vi "Robot Movement Command Interpreter-poly.vi"   [LabVIEW 2019]
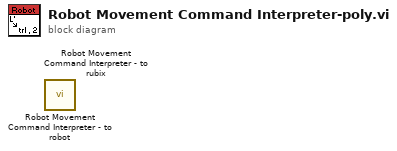
[diagram p0: block diagram]
diagram:
  n1 = call "Robot Movement Command Interpreter - to robot.vi"() -> ()  [unwired: 11 in, 1 out]
  n2 = call "Robot Movement Command Interpreter - to rubix.vi"() -> ()  [unwired: 9 in, 3 out]
